vi "HEIDOLPH_CONTROL09.vi"(6 "master":bool, 7 "Array":dbl[](array[numeric]), 8 "shutdown":bool, 9 "Bypass select":enum32{"Remote", "Manual"}(radio), 10 "Set RPM":dbl(slide) scale=0.0..500.0, 11 "Device port":dbl=13.0) -> (1 "Dynamic Data":dynamicdata(waveform), 2 "RPM":dbl, 3 "RPM 2":dbl, 4 "Torque":dbl, 5 "Torque 2":dbl)   [LabVIEW 2015]
uses:
  x64/Debug/BERTTA.dll
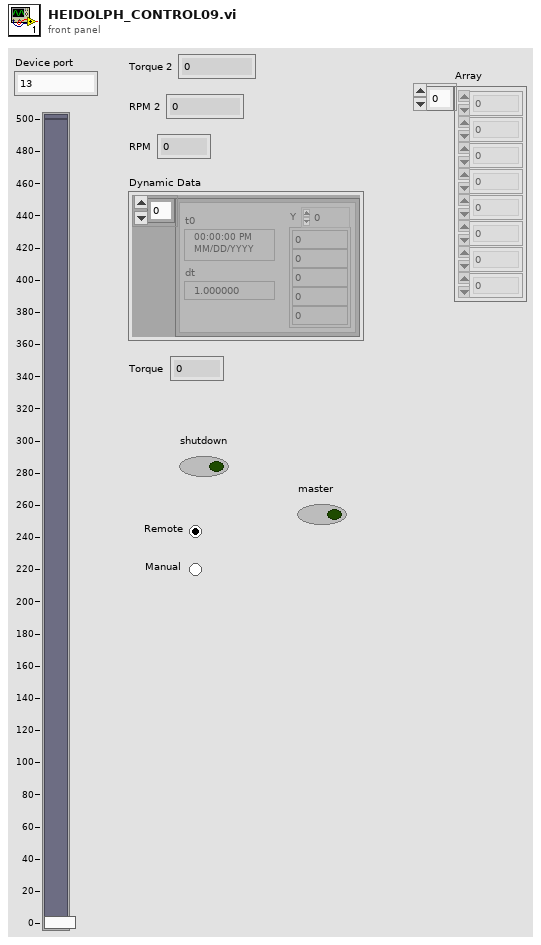
[diagram p1: front panel]
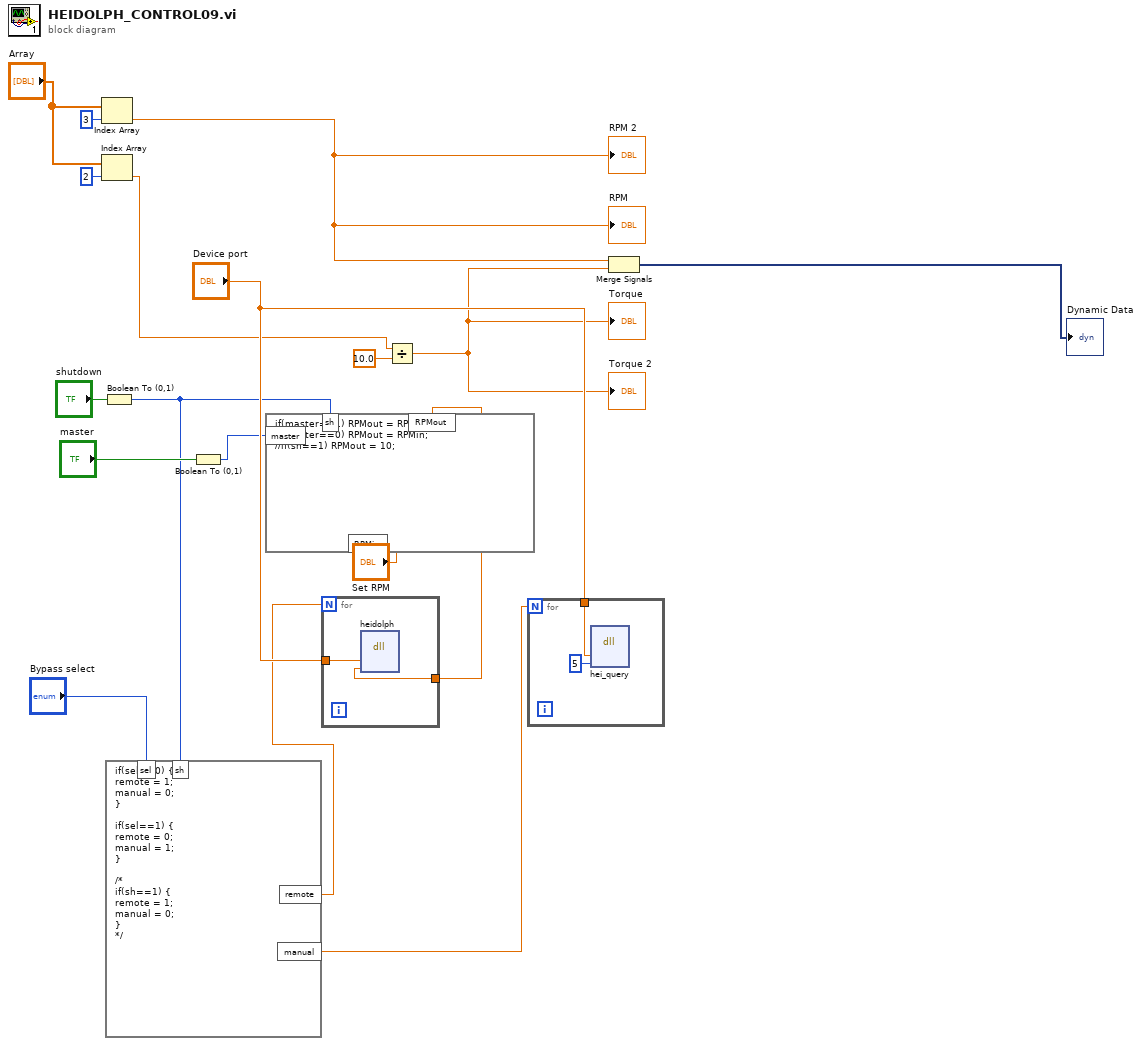
[diagram p0: block diagram]
diagram:
  n1 = Index Array(array="Array", index=3) -> (element=w2:dbl)
  "RPM" <- w2
  "RPM 2" <- w2
  n2 = Index Array(array="Array", index=2) -> (element=w1:dbl)
  n3 = Boolean To (0,1)(Boolean="shutdown") -> (0, 1=w8:i16)
  n4 = formula code="if(sel==0) {\nremote = 1;\nmanual = 0;\n}\n\nif(sel==1) {\nremote = 0;\nmanual = 1;\n}\n\n/*\nif(sh==1) {\nremote = 1;\nmanual = 0;\n}\n*/"("sel"="Bypass select", "sh"=w8) -> ("remote"=w13:dbl, "manual"=w12:dbl)
  n5 = Boolean To (0,1)(Boolean="master") -> (0, 1=w9:i16)
  n6 = formula code="if(master==1) RPMout = RPMin;\nif(master==0) RPMout = RPMin;\n//if(sh==1) RPMout = 10;"("sh"=w8, "RPMin"="Set RPM", "master"=w9) -> ("RPMout"=w16:dbl)
  n7 = for {
    N: w13 -> [_]
    tunnel: w16 -> [w20]
    tunnel: "Device port" -> [w19]
    n8 = dll-call lib="C:/Users/shresplab/OneDrive - Kemira Oyj/Documents/Visual Studio 2017/Projects/Bertta/BERTTA/x64/Debug/BERTTA.dll" fn="heidolph"("port"=w19, "speed"=w20) -> ()  [unwired: 6 in, 2 out]
  }
  n9 = Divide(x=w1, y=10.0) -> (x/y=w7:dbl)
  "Torque" <- w7
  "Torque 2" <- w7
  n10 = for {
    N: w12 -> [_]
    tunnel: "Device port" -> [w22]
    n11 = dll-call lib="C:/Users/shresplab/OneDrive - Kemira Oyj/Documents/Visual Studio 2017/Projects/Bertta/BERTTA/x64/Debug/BERTTA.dll" fn="hei_query"("port"=w22, "q"=5) -> ()  [unwired: 6 in, 2 out]
  }
  n12 = Merge Signals(w2, w7) -> (→"Dynamic Data":dynamicdata)
